vi "transfer char run_subvi_7_25_12c_JW.vi"(0 "VISA session":refnum<visa-resource-name>="GPIB0::17::INSTR", 5 "Var1 sweep settings":T6={"start"=40.0, "stop"=-40.0, "step (linear only)"=-1.0, "sweep spacing (linear: 0)"=0, "sweep mode"=FALSE, "compliance (V)"=100.0, "compliance (A)"=0.001} {"compliance (A)" format="%^.2e"; "compliance (V)" format="%.2f"; "sweep spacing (linear: 0)" items=["linear", "log 10", "log 25", "log 50"]; "step (linear only)" format="%.2f"; "stop" format="%.2f"; "start" format="%.2f"}, 7 "Var2 step settings":T5={"compliance (A)"=0.001, "compliance (V)"=100.0, "start"=-2.0, "total points"=2, "step"=-38.0} {"step" format="%.2f"; "start" format="%.2f"; "compliance (V)" format="%.2f"; "compliance (A)" format="%^.2e"}, 9 "integration time":u32(slide) scale=0.0..2.0, 11 "Input Path":path, 13 "Sample Properties:":T3 {"Date Created" format="%<%x>T"}) -> (2 "Check Cluster":T1, 4 "Output":T2 {"Mobility-Lin" format="%#_4e"; "Mobility-Sat" format="%#_4e"}, 6 "graphic display":cluster{"trace":dbl[], "trace":dbl[]}(graph), 8 "Log Plot":cluster{dbl[], dbl[]}(graph), 10 "XY Graph":cluster{dbl[], "trace":dbl[]}[](graph), 14 "Raw Graph":cluster{dbl[], dbl[]}[](graph), 15 "error?":errorcluster)   [LabVIEW 2011]
uses:
  <vilib>/Utility/file.llb/Write To Spreadsheet File (DBL).vi
panel:
  out "Test Array 2":string[][](array[string])
  out "Test Array":dbl[](array[numeric])
  in  "Output Path":path
  in  "Temp (K)":dbl=0.001 format="%^.2e"
  in  "NumPts":dbl=5.0
  out "Numeric":dbl
  out "min r":dbl
  out "max r":dbl
  out "error? 2":errorcluster
  in  "MAXIMUM":ext format="%.2e"
  in  "MINIMUM":ext=-1e-05 format="%_2e"
  out "graphic display 2":cluster{"trace":dbl[], "trace":dbl[]}(graph)
  in  "Y1 axis":string="Id"
  in  "Y2 axis settings":T4 {"MAXIMUM" format="%.9f"; "MINIMUM" format="%.9f"}
  in  "wait time parameter":dbl=1.0
  in  "Value (Either V or A) 4":dbl
  in  "Value (Either V or A) 3":dbl
  in  "Value (Either V or A) 2":dbl
  in  "Value (V or A)":dbl
  in  "compliance (A)":dbl=0.001 format="%^.2e"
  in  "compliance (V)":dbl=100.0 format="%^.2e"
  in  "Iname":string="Is"
  in  "Vname":string="Vs"
  in  "Function":u16(ring)=4 items=["disabled", "Var1", "Var2", "Var1'", "Constant"]
  in  "Mode":u16(ring)=4 items=["V", "I", "VPulse", "IPulse", "Common"]
  in  "Iname 4":string="I4"
  in  "Vname 4":string="V4"
  in  "Function 4":u16(ring)=4 items=["disabled", "Var1", "Var2", "Var1'", "Constant"]
  in  "Mode 4":u16(ring) items=["V", "I", "VPulse", "IPulse", "Common"]
  in  "Iname 3":string="Ig"
  in  "Vname 3":string="Vg"
  in  "Function 3":u16(ring)=1 items=["disabled", "Var1", "Var2", "Var1'", "Constant"]
  in  "Mode 3":u16(ring) items=["V", "I", "VPulse", "IPulse", "Common"]
  in  "Iname 2":string="Id"
  in  "Vname 2":string="Vd"
  in  "Function 2":u16(ring)=2 items=["disabled", "Var1", "Var2", "Var1'", "Constant"]
  in  "Mode 2":u16(ring) items=["V", "I", "VPulse", "IPulse", "Common"]
  in  "reset":bool=TRUE
  # "SMU1"
  # "SMU2"
  # "SMU3"
  # "SMU4"
  # "Sample Properties:"
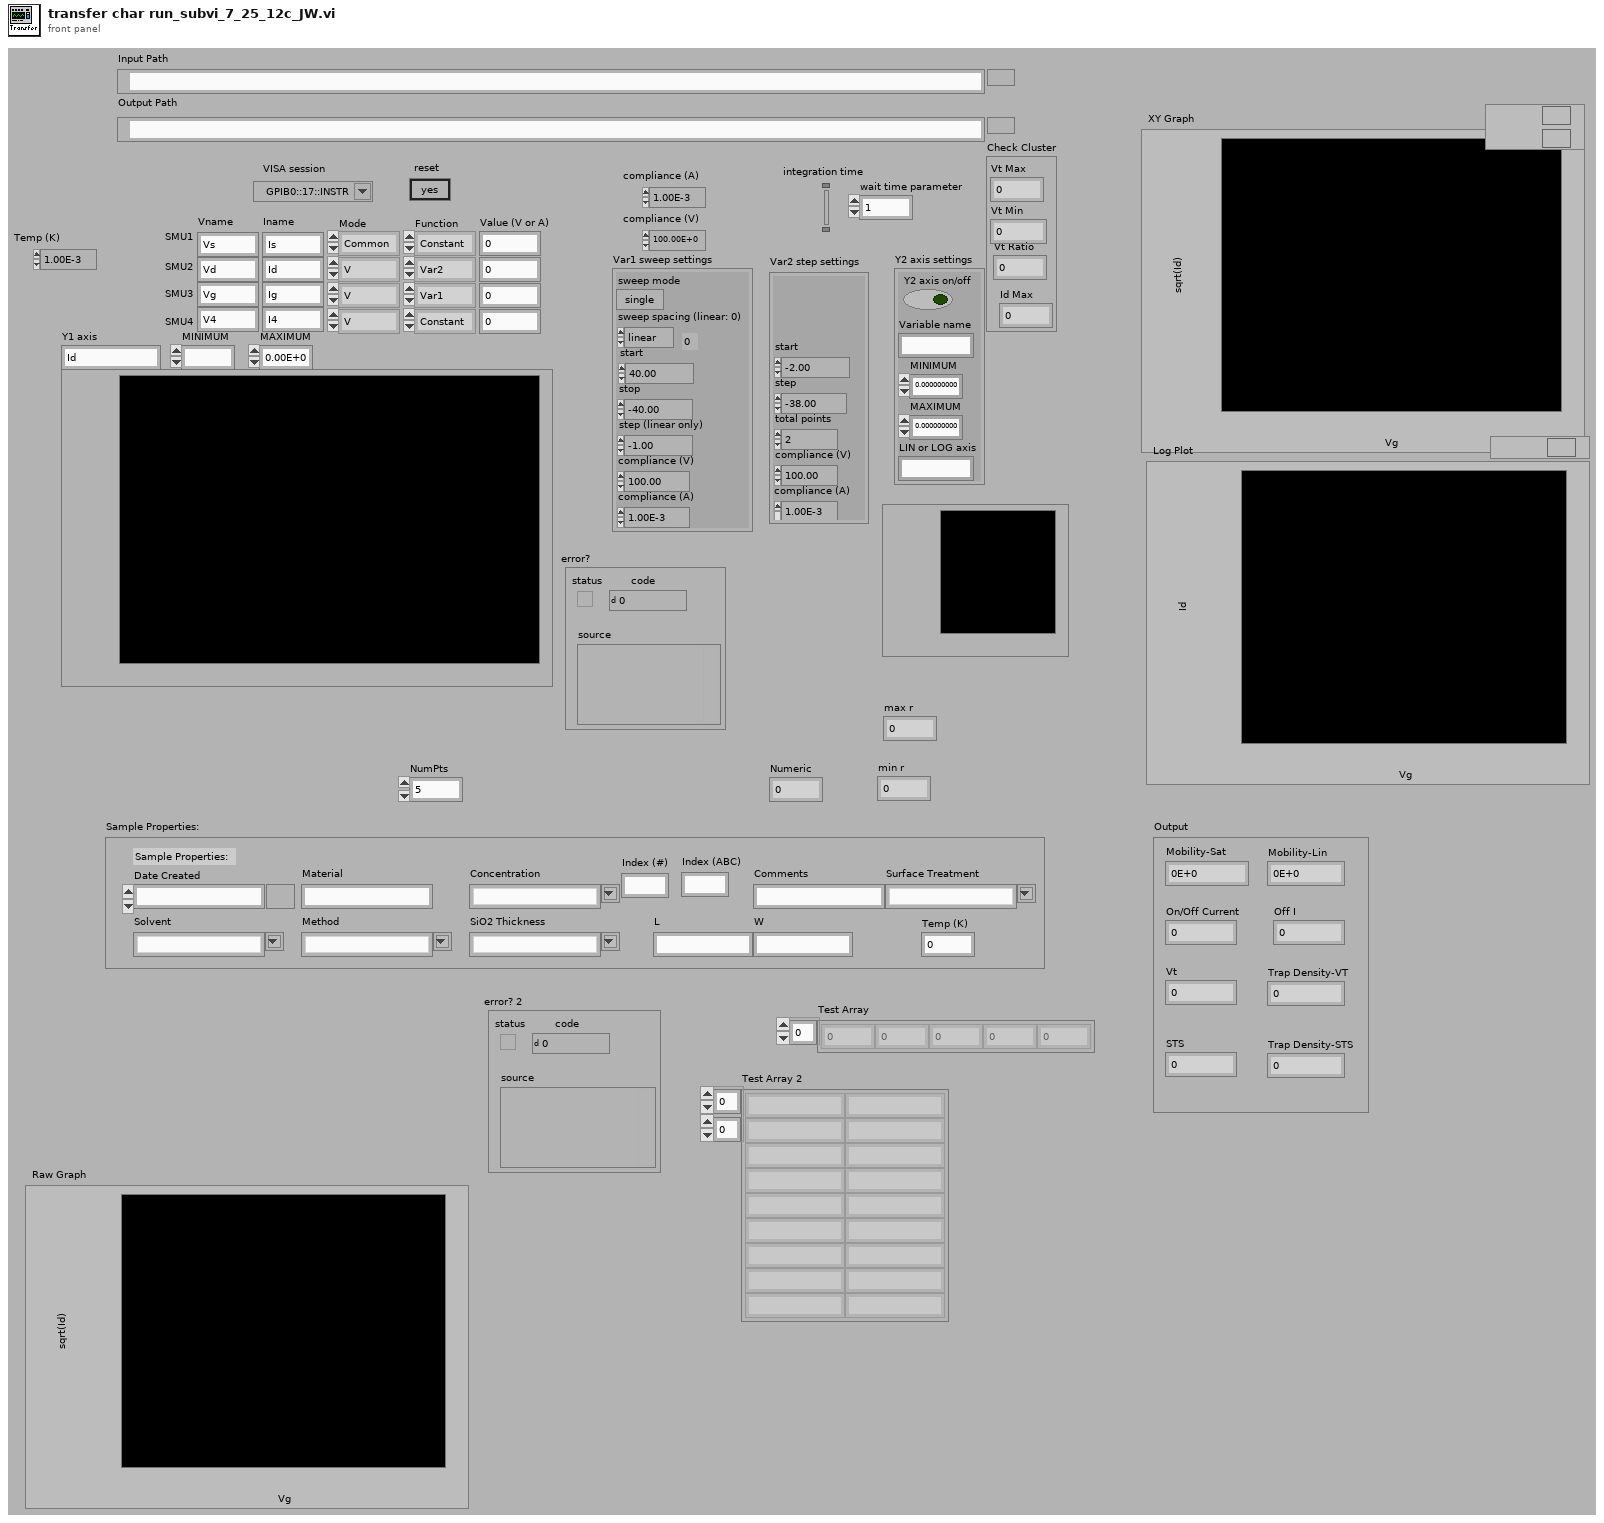
[diagram p1: front panel]
types:
  T1 = cluster{"Vt Max":i32, "Vt Min":i32, "Vt Ratio":i32, "Id Max":dbl}
  T2 = cluster{"Mobility-Sat":dbl, "Mobility-Lin":dbl, "On/Off Current":dbl, "Off I":dbl, "Vt":dbl, "STS":dbl, "Trap Density-VT":dbl, "Trap Density-STS":dbl}
  T3 = cluster{"Date Created":timestamp, "Material":string, "Solvent":string, "Concentration":string, "Method":string, "SiO2 Thickness":string, "Index (#)":string, "Index (ABC)":string, "L":string, "W":string, "Surface Treatment":string, "Comments":string, "Temp (K)":dbl}
  T4 = cluster{"Y2 axis on/off":bool, "MINIMUM":ext, "MAXIMUM":ext, "Variable name":string, "LIN or LOG axis":string}
  T5 = cluster{"compliance (A)":dbl, "compliance (V)":dbl, "start":dbl, "total points":u16, "step":dbl}
  T6 = cluster{"start":dbl, "stop":dbl, "step (linear only)":dbl, "sweep spacing (linear: 0)":u16, "sweep mode":bool, "compliance (V)":dbl, "compliance (A)":dbl}
  T7 = cluster{"Vt Max":dbl, "Vt Min":dbl, "Vt Ratio":dbl, "Id Max":dbl}
  T8 = cluster{"Mobility-Sat":dbl, "Mobility-Lin":dbl, "On/Off I-Sat":dbl, "Off I-Sat":dbl, "VT-Sat":dbl, "Sub Threshold Swing":dbl, "Trap Density-VT":dbl, "Trap Density (N)":dbl}
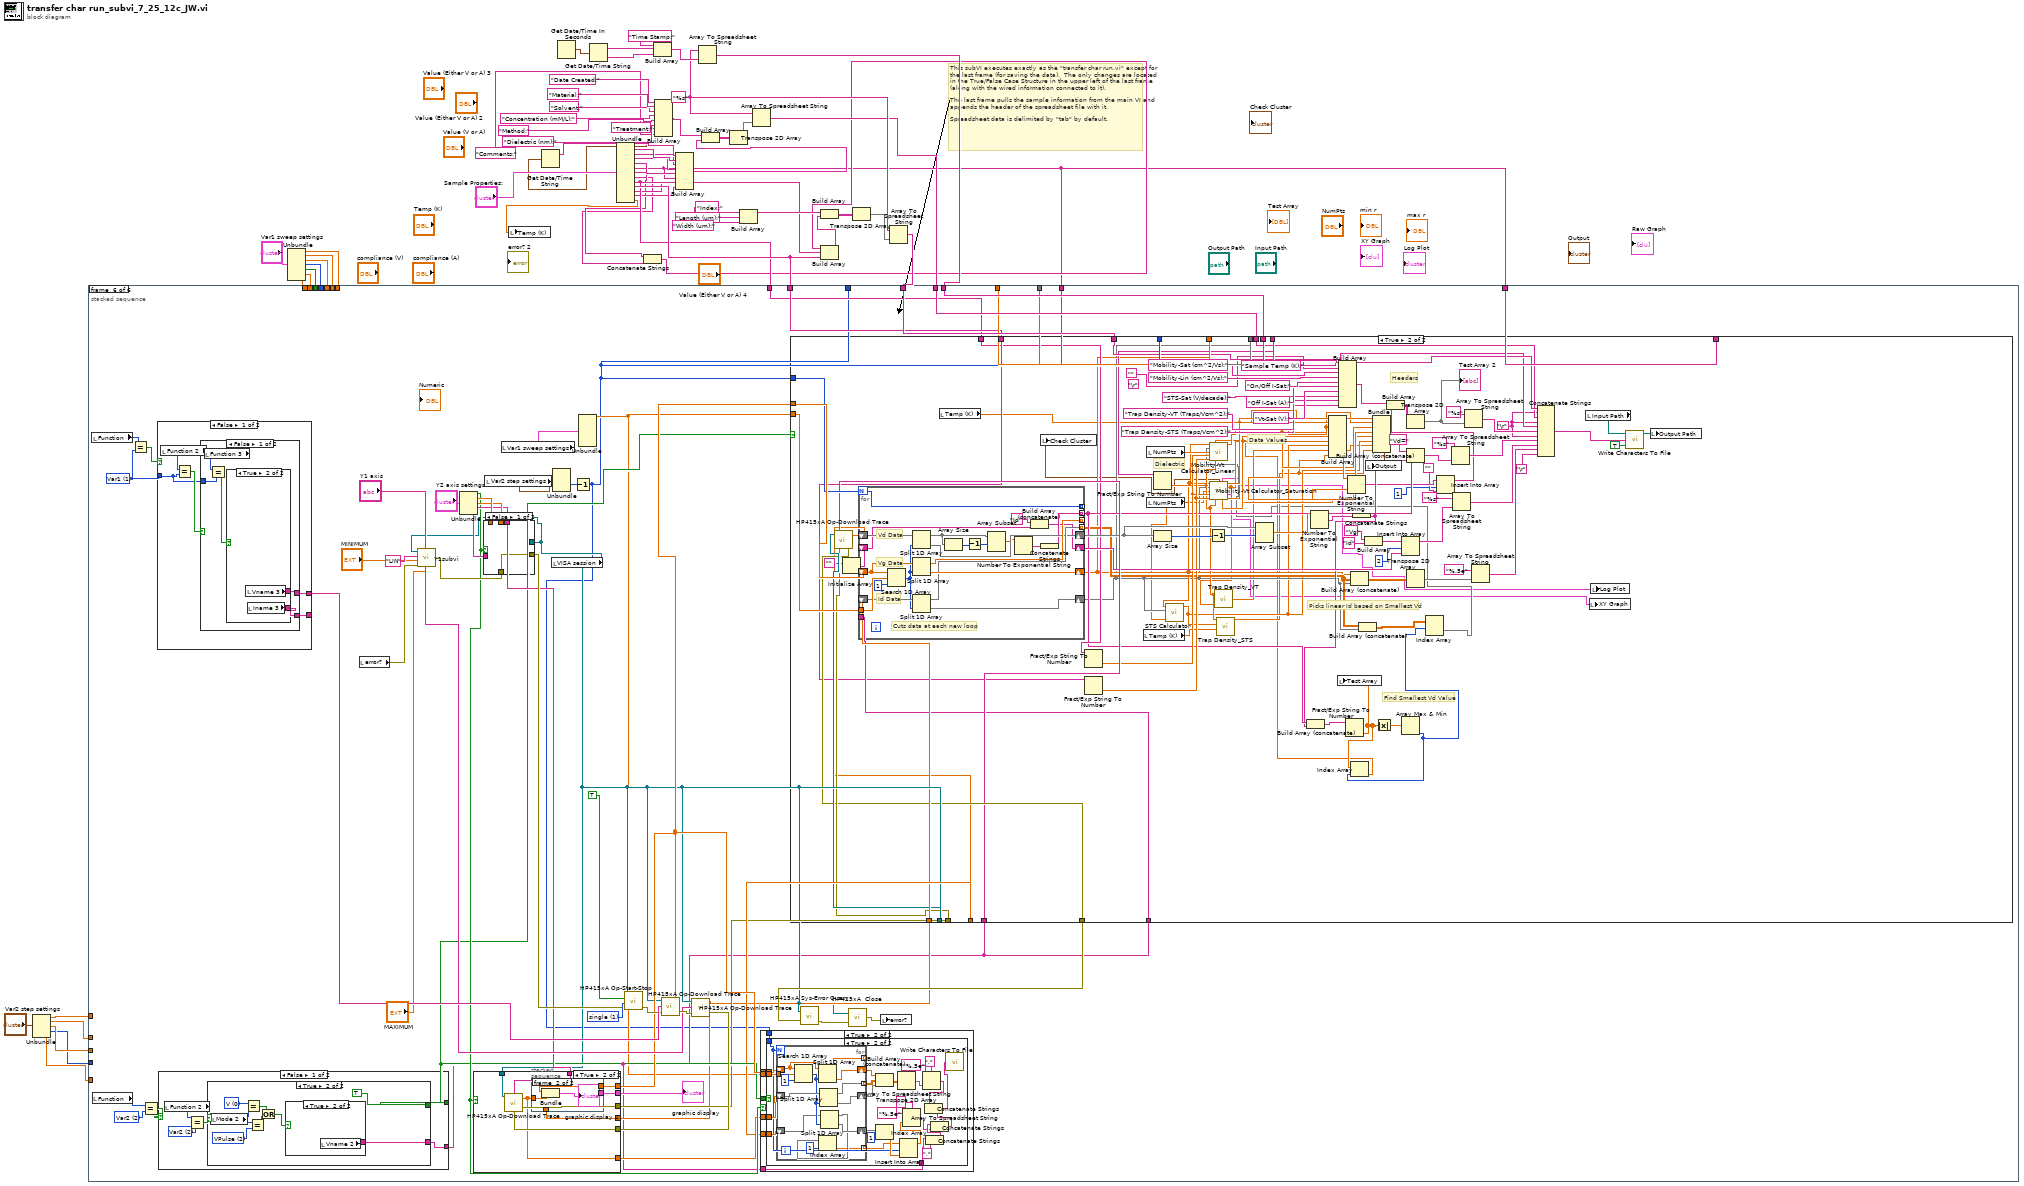
[diagram p0: block diagram]
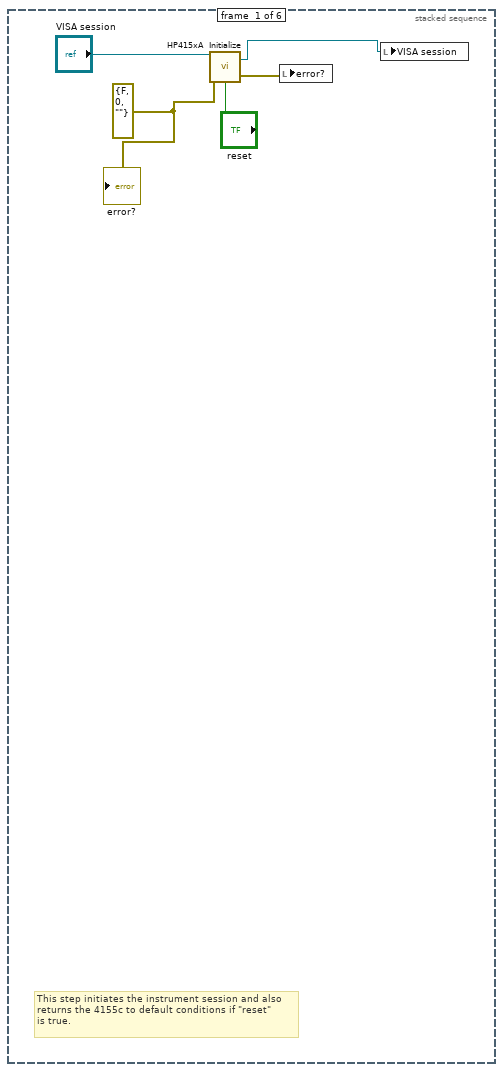
[diagram p2: hidden frame]
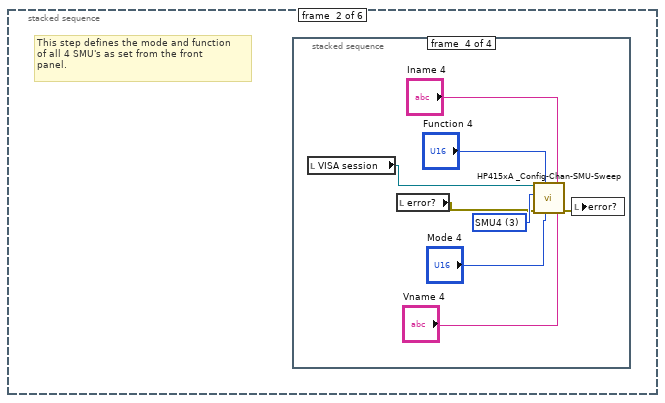
[diagram p3: hidden frame]
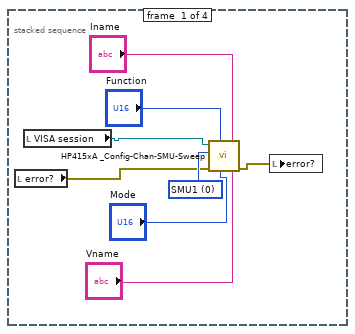
[diagram p4: hidden frame]
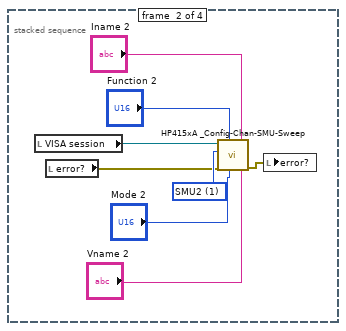
[diagram p5: hidden frame]
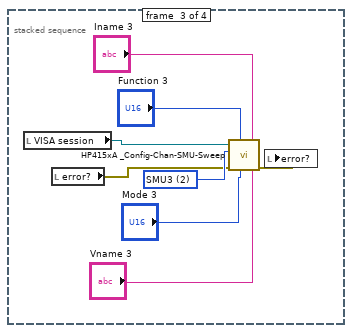
[diagram p6: hidden frame]
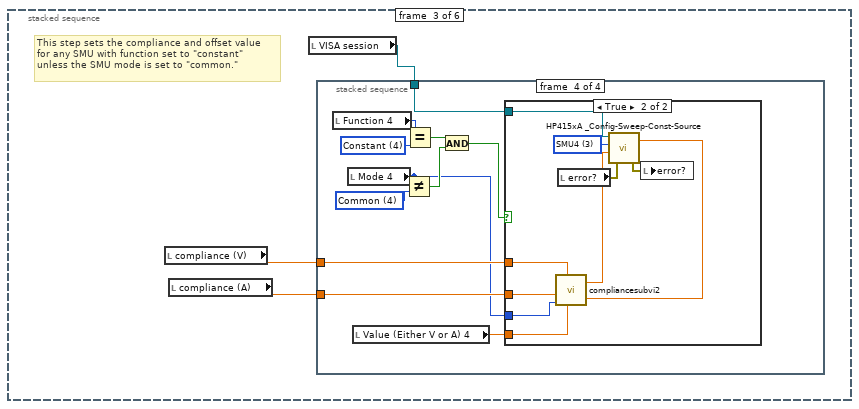
[diagram p7: hidden frame]
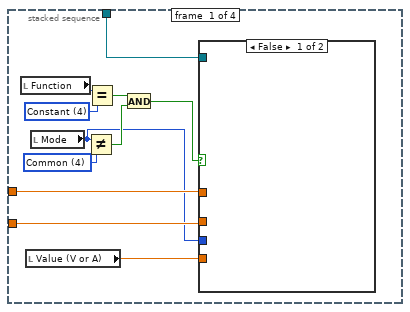
[diagram p8: hidden frame]
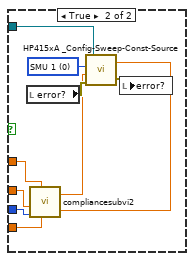
[diagram p9: hidden frame]
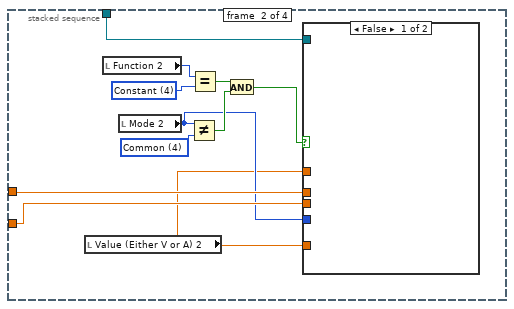
[diagram p10: hidden frame]
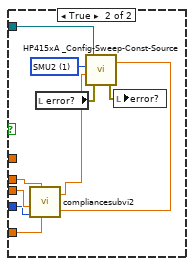
[diagram p11: hidden frame]
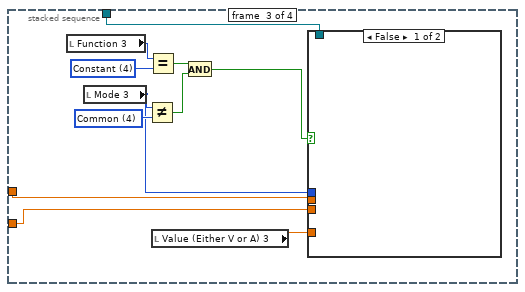
[diagram p12: hidden frame]
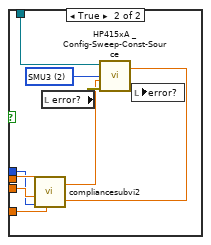
[diagram p13: hidden frame]
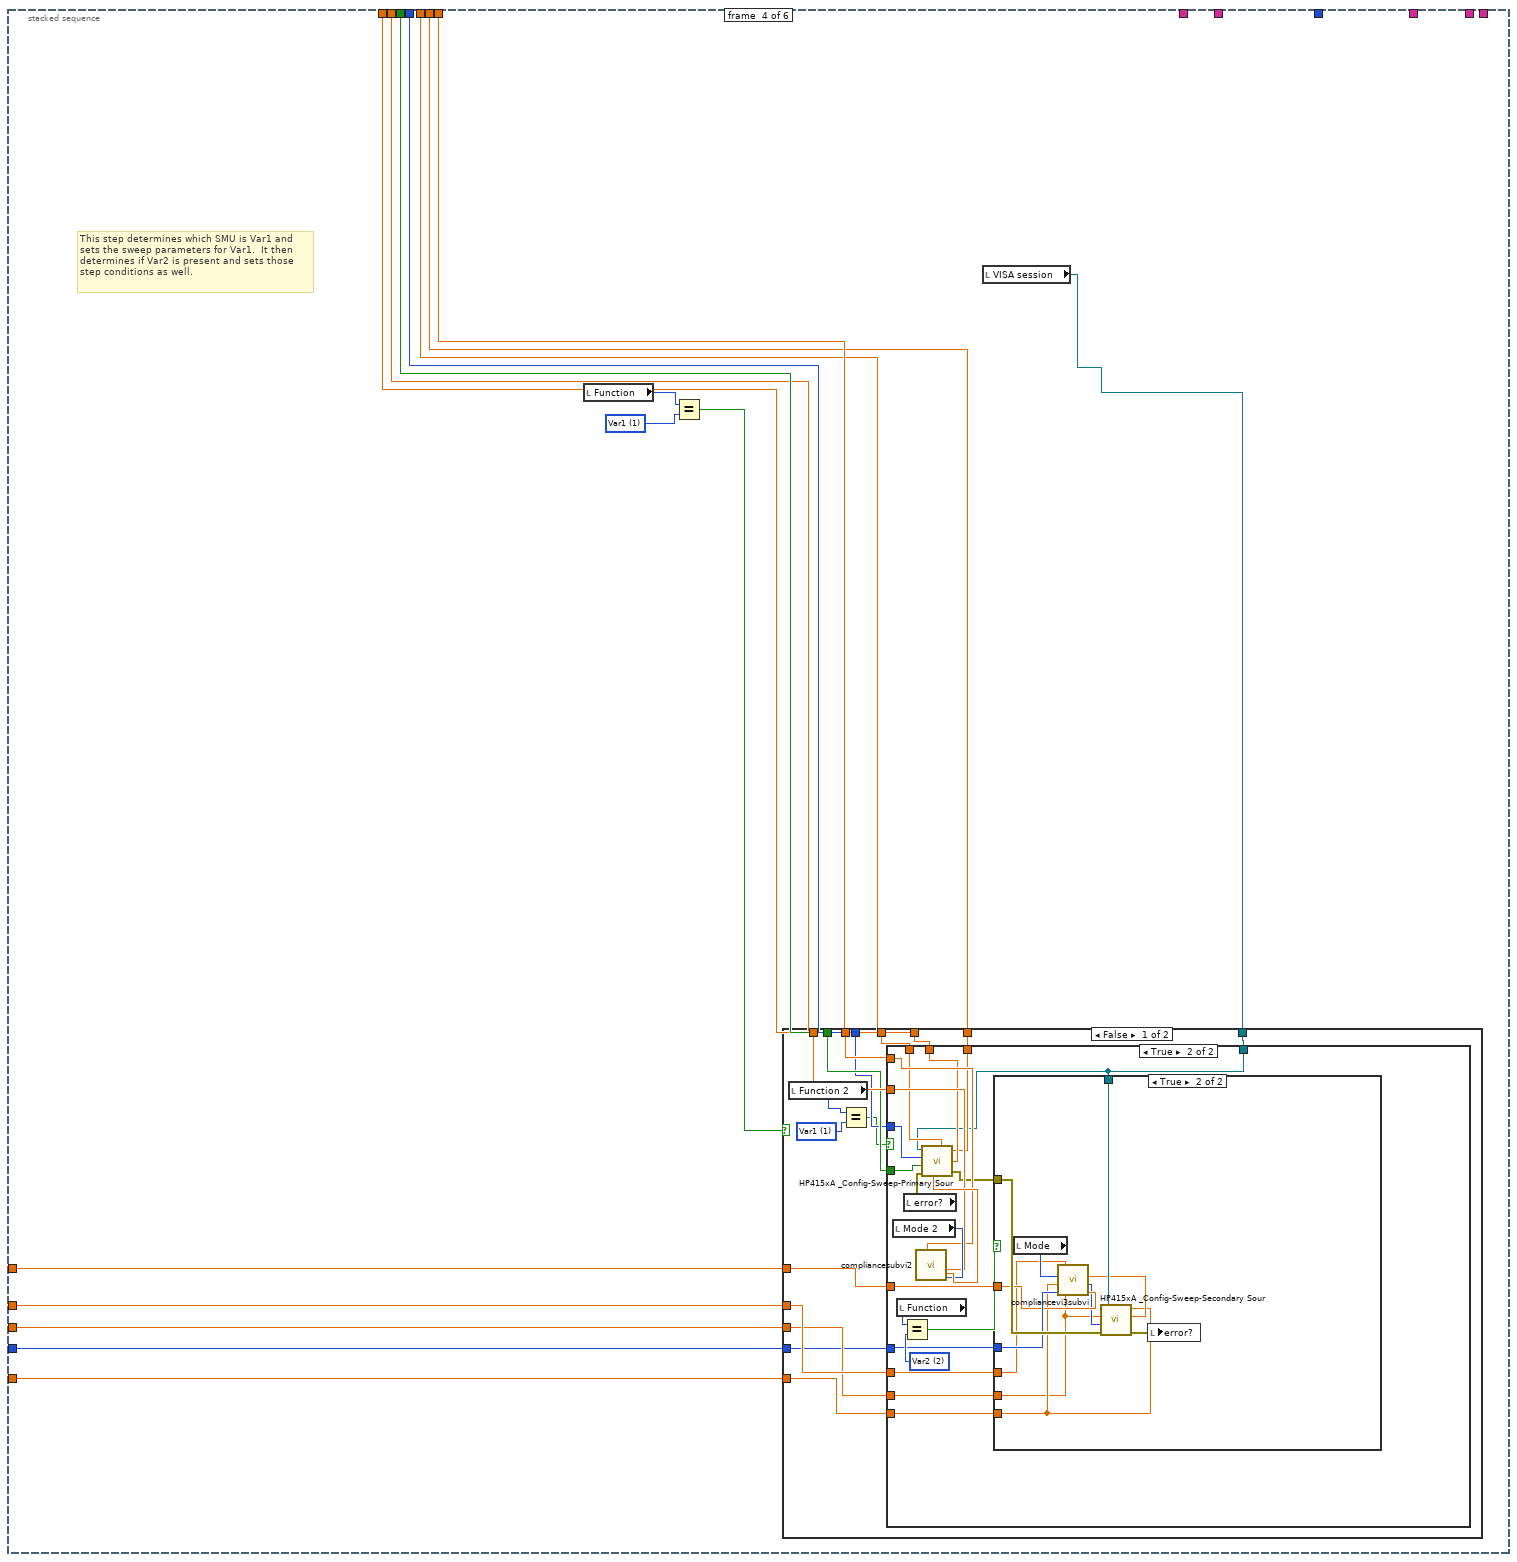
[diagram p15: hidden frame]
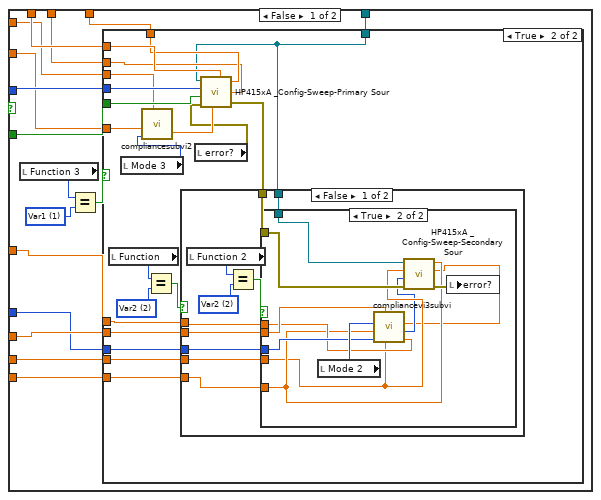
[diagram p16: hidden frame]
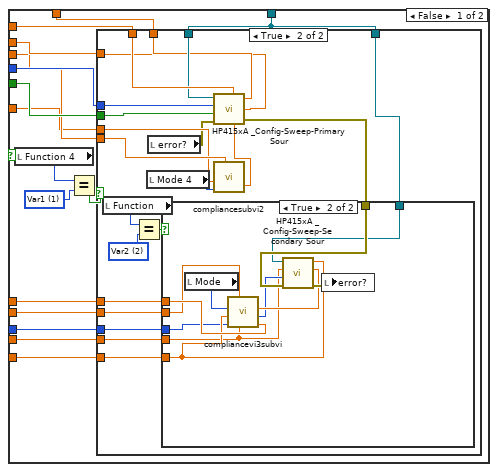
[diagram p17: hidden frame]
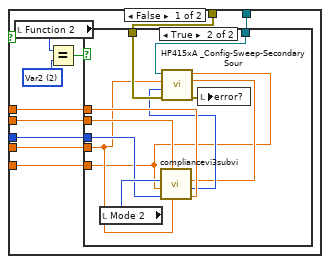
[diagram p19: hidden frame]
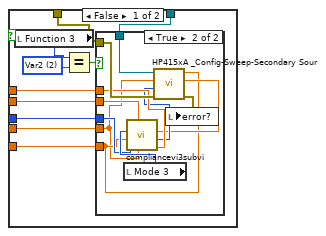
[diagram p20: hidden frame]
diagram:
  w31 = "%s"
  # "This subVI executes exactly as the \"transfer char run.vi\" except for the last frame (for saving the data).  The only changes are located in the True/False Case Structure in the upper left of the last frame (along with the wired information connected to it). \n\nThe last frame pulls the sample information from the main VI and appends the header of the spreadsheet file with it.\n\nSpreadsheet data is delimited by \"tab\" by default."
  n1 = Unbundle("Var2 step settings") -> ("compliance (A)"=w49:dbl, "compliance (V)"=w48:dbl, "start"=w47:dbl, "total points"=w46:u16, "step"=w45:dbl)
  n2 = Unbundle("Var1 sweep settings") -> ("start"=w57:dbl, "stop"=w56:dbl, "step (linear only)"=w55:dbl, "sweep spacing (linear: 0)"=w54:u16, "sweep mode"=w53:bool, "compliance (V)"=w52:dbl, "compliance (A)"=w51:dbl)
  n3 = Get Date/Time In Seconds() -> (seconds since 1Jan1904=w38:timestamp)
  n4 = Get Date/Time String(seconds (now)=w38) -> (date string=w37:string, time string=w36:string)  [unwired: 2 in]
  n5 = Unbundle("Sample Properties:") -> ("Date Created"=w16:timestamp, "Material"=w15:string, "Solvent"=w11:string, "Concentration"=w10:string, "Method"=w14:string, "SiO2 Thickness"=w1:string, "Index (#)"=w5:string, "Index (ABC)"=w4:string, "L"=w8:string, "W"=w9:string, "Surface Treatment"=w7:string, "Comments"=w6:string, "Temp (K)"=w2:dbl)
  n6 = local write "Temp (K)"(w2) -> ()
  n7 = Get Date/Time String(seconds (now)=w16) -> (date string=w43:string)  [unwired: 2 in, 1 out]
  n8 = Concatenate Strings(w5, w4) -> (w3:string)
  n9 = Build Array("Time Stamp:", w37, w36) -> (w35:string[])
  n10 = Build Array("Date Created:", "Material:", "Solvent:", "Concentration (mM/L):", "Method:", "Dielectric (nm):", "Treatment:", "Comments:") -> (w26:string[])
  n11 = Build Array(w43, w15, w11, w10, w14, w1, w7, w6) -> (w25:string[])
  n12 = Array To Spreadsheet String(array=w35, 3:w31) -> (spreadsheet string=w27:string)  [unwired: 1 in]
  n13 = Build Array(w26, w25) -> (w24:string[][])
  n14 = Transpose 2D Array(2D array=w24) -> (transposed array=w23:string[][])
  n15 = Build Array("Index:", "Length (um):", "Width (um):") -> (w22:string[])
  n16 = Array To Spreadsheet String(array=w23, 3:w31) -> (spreadsheet string=w30:string)  [unwired: 1 in]
  n17 = Build Array(w3, w8, w9) -> (w21:string[])
  n18 = Build Array(w22, w21) -> (w20:string[][])
  n19 = Transpose 2D Array(2D array=w20) -> (transposed array=w19:string[][])
  n20 = Array To Spreadsheet String(array=w19, 3:w31) -> (spreadsheet string=w18:string)  [unwired: 1 in]
  n21 = stacked-sequence {
    tunnel: w57 -> [_ _ _ w194 _ _]
    tunnel: w56 -> [_ _ _ w193 _ _]
    tunnel: w55 -> [_ _ _ w192 _ _]
    tunnel: w54 -> [_ _ _ w191 _ _]
    tunnel: w53 -> [_ _ _ w190 _ _]
    tunnel: w52 -> [_ _ _ w189 _ _]
    tunnel: w51 -> [_ _ _ w188 _ _]
    tunnel: w49 -> [_ _ _ w187 _ _]
    tunnel: w48 -> [_ _ _ w186 _ _]
    tunnel: w47 -> [_ _ _ w185 _ _]
    tunnel: w46 -> [_ _ _ w184 _ _]
    tunnel: w45 -> [_ _ _ w183 _ _]
    tunnel: w27 -> [_ _ _ _ _ w558]
    tunnel: w30 -> [_ _ _ _ _ w557]
    tunnel: w18 -> [_ _ _ _ _ w556]
    tunnel: [_ _ _ _ _ w555] -> _
    tunnel: [_ _ _ _ _ w554] -> _
    tunnel: [_ _ _ _ _ w551] -> _
    tunnel: w9 -> [_ _ _ _ _ w553]
    tunnel: w8 -> [_ _ _ _ _ w552]
    tunnel: w1 -> [_ _ _ _ _ w550]
    tunnel: w1 -> [_ _ _ _ _ w549]
    frame #0 {
      w62 = errorcluster {"status"=FALSE, "code"=0, "source"=""} ("error out")
      # "This step initiates the instrument session and also\nreturns the 4155c to default conditions if \"reset\"\nis true."
      n22 = call "HP415xA  Initialize.vi"("instrument descriptor"="VISA session", "reset"="reset", "error in (no error)"=w62) -> ("VISA session"=w59:refnum<visa-resource-name>, "error out"=w61:errorcluster)  [unwired: 2 in]
      n23 = local write "error?"(w61) -> ()
      n24 = local write "VISA session"(w59) -> ()
      "error?" <- w62
    }
    frame #1 {
      # "This step defines the mode and function\nof all 4 SMU's as set from the front\npanel."
      n25 = stacked-sequence {
        frame #0 {
          w71 = u32 0 items=["SMU1  ", "SMU2  ", "SMU3  ", "SMU4  ", "SMU5  ", "SMU6  "] ("unit to configure")
          n26 = local read "error?"() -> (w66:errorcluster)
          n27 = local read "VISA session"() -> (w64:refnum<visa-resource-name>)
          n28 = call "HP415xA _Config-Chan-SMU-Sweep.vi"("V name (max 6 chars)"="Vname", "I name (max 6 chars)"="Iname", "mode"="Mode", "function"="Function", "error in (no error)"=w66, "unit to configure"=w71, "VISA session"=w64) -> ("error out"=w65:errorcluster)  [unwired: 2 in]
          n29 = local write "error?"(w65) -> ()
        }
        frame #1 {
          w75 = u32 1 items=["SMU1  ", "SMU2  ", "SMU3  ", "SMU4  ", "SMU5  ", "SMU6  "] ("unit to configure")
          n30 = local read "VISA session"() -> (w72:refnum<visa-resource-name>)
          n31 = local read "error?"() -> (w73:errorcluster)
          n32 = call "HP415xA _Config-Chan-SMU-Sweep.vi"("V name (max 6 chars)"="Vname 2", "I name (max 6 chars)"="Iname 2", "mode"="Mode 2", "function"="Function 2", "error in (no error)"=w73, "unit to configure"=w75, "VISA session"=w72) -> ("error out"=w74:errorcluster)  [unwired: 2 in]
          n33 = local write "error?"(w74) -> ()
        }
        frame #2 {
          w83 = u32 2 items=["SMU1  ", "SMU2  ", "SMU3  ", "SMU4  ", "SMU5  ", "SMU6  "] ("unit to configure")
          n34 = local read "VISA session"() -> (w80:refnum<visa-resource-name>)
          n35 = local read "error?"() -> (w81:errorcluster)
          n36 = call "HP415xA _Config-Chan-SMU-Sweep.vi"("V name (max 6 chars)"="Vname 3", "I name (max 6 chars)"="Iname 3", "mode"="Mode 3", "function"="Function 3", "error in (no error)"=w81, "unit to configure"=w83, "VISA session"=w80) -> ("error out"=w82:errorcluster)  [unwired: 2 in]
          n37 = local write "error?"(w82) -> ()
        }
        frame #3 {
          w91 = u32 3 items=["SMU1  ", "SMU2  ", "SMU3  ", "SMU4  ", "SMU5  ", "SMU6  "] ("unit to configure")
          n38 = local read "VISA session"() -> (w88:refnum<visa-resource-name>)
          n39 = local read "error?"() -> (w90:errorcluster)
          n40 = call "HP415xA _Config-Chan-SMU-Sweep.vi"("V name (max 6 chars)"="Vname 4", "I name (max 6 chars)"="Iname 4", "mode"="Mode 4", "function"="Function 4", "error in (no error)"=w90, "unit to configure"=w91, "VISA session"=w88) -> ("error out"=w89:errorcluster)  [unwired: 2 in]
          n41 = local write "error?"(w89) -> ()
        }
      }
    }
    frame #2 {
      # "This step sets the compliance and offset value\nfor any SMU with function set to \"constant\"\nunless the SMU mode is set to \"common.\""
      n42 = local read "compliance (V)"() -> (w97:dbl)
      n43 = local read "compliance (A)"() -> (w98:dbl)
      n44 = local read "VISA session"() -> (w96:refnum<visa-resource-name>)
      n45 = stacked-sequence {
        tunnel: w96 -> [w107 w127 w146 w166]
        tunnel: w98 -> [w101 w123 w144 w164]
        tunnel: w97 -> [w100 w122 w143 w165]
        frame #0 {
          w105 = u16 4 items=["V", "I", "VPulse", "IPulse", "Common"] ("Mode")
          w109 = u16 4 items=["disabled", "Var1", "Var2", "Var1'", "Constant"] ("Function")
          n46 = local read "Function"() -> (w108:u16)
          n47 = local read "Value (V or A)"() -> (w102:dbl)
          n48 = local read "Mode"() -> (w99:u16)
          n49 = Not Equal?(x=w99, y=w105) -> (x != y?=w104:bool)
          n50 = Equal?(x=w108, y=w109) -> (x = y?=w106:bool)
          n51 = And(x=w106, y=w104) -> (x .and. y?=w103:bool)
          n52 = case shown="False" w103 {
            tunnel: w107 -> [_ w119]
            tunnel: w100 -> [_ w115]
            tunnel: w101 -> [_ w114]
            tunnel: w102 -> [_ w111]
            tunnel: w99 -> [_ w112]
            frame False {
            }
            frame True {
              w118 = u16 0 items=["SMU 1", "SMU2", "SMU3", "SMU4", "SMU5", "SMU6", "VSU1", "VSU2"] ("unit (SMU1:0)")
              n53 = local read "error?"() -> (w117:errorcluster)
              n54 = call "compliancesubvi2.vi"("Value1"=w111, "compliance (V)"=w115, "Mode"=w112, "compliance (A)"=w114) -> ("compliance"=w113:dbl, "constant"=w110:dbl)  [unwired: 2 in]
              n55 = call "HP415xA _Config-Sweep-Const-Source.vi"("compliance (SMUs only)"=w113, "error in (no error)"=w117, "source (V or A)"=w110, "unit (SMU1:0)"=w118, "VISA session"=w119) -> ("error out"=w116:errorcluster)
              n56 = local write "error?"(w116) -> ()
            }
          }
        }
        frame #1 {
          w124 = u16 4 items=["V", "I", "VPulse", "IPulse", "Common"] ("Mode 2")
          w125 = u16 4 items=["disabled", "Var1", "Var2", "Var1'", "Constant"] ("Function 2")
          n57 = local read "Value (Either V or A) 2"() -> (w120:dbl)
          n58 = local read "Function 2"() -> (w126:u16)
          n59 = local read "Mode 2"() -> (w121:u16)
          n60 = Not Equal?(x=w121, y=w124) -> (x != y?=w129:bool)
          n61 = Equal?(x=w126, y=w125) -> (x = y?=w130:bool)
          n62 = And(x=w130, y=w129) -> (x .and. y?=w128:bool)
          n63 = case shown="False" w128 {
            tunnel: w127 -> [_ w140]
            tunnel: w122 -> [_ w138]
            tunnel: w123 -> [_ w137]
            tunnel: w120 -> [_ _]
            tunnel: w121 -> [_ w133]
            tunnel: w120 -> [_ w132]
            frame False {
            }
            frame True {
              w139 = u16 1 items=["SMU 1", "SMU2", "SMU3", "SMU4", "SMU5", "SMU6", "VSU1", "VSU2"] ("unit (SMU1:0)")
              n64 = call "compliancesubvi2.vi"("Value1"=w132, "compliance (V)"=w138, "Mode"=w133, "compliance (A)"=w137) -> ("compliance"=w136:dbl, "constant"=w131:dbl)  [unwired: 2 in]
              n65 = local read "error?"() -> (w135:errorcluster)
              n66 = call "HP415xA _Config-Sweep-Const-Source.vi"("compliance (SMUs only)"=w136, "error in (no error)"=w135, "source (V or A)"=w131, "unit (SMU1:0)"=w139, "VISA session"=w140) -> ("error out"=w134:errorcluster)
              n67 = local write "error?"(w134) -> ()
            }
          }
        }
        frame #2 {
          w148 = u16 4 items=["V", "I", "VPulse", "IPulse", "Common"] ("Mode 2")
          w149 = u16 4 items=["disabled", "Var1", "Var2", "Var1'", "Constant"] ("Function 2")
          n68 = local read "Function 3"() -> (w147:u16)
          n69 = local read "Mode 3"() -> (w142:u16)
          n70 = Not Equal?(x=w142, y=w148) -> (x != y?=w150:bool)
          n71 = Equal?(x=w147, y=w149) -> (x = y?=w151:bool)
          n72 = local read "Value (Either V or A) 3"() -> (w145:dbl)
          n73 = And(x=w151, y=w150) -> (x .and. y?=w141:bool)
          n74 = case shown="False" w141 {
            tunnel: w146 -> [_ w159]
            tunnel: w145 -> [_ w153]
            tunnel: w144 -> [_ w156]
            tunnel: w143 -> [_ w155]
            tunnel: w142 -> [_ w154]
            frame False {
            }
            frame True {
              w158 = u16 2 items=["SMU 1", "SMU2", "SMU3", "SMU4", "SMU5", "SMU6", "VSU1", "VSU2"] ("unit (SMU1:0)")
              n75 = call "compliancesubvi2.vi"("Value1"=w153, "compliance (V)"=w155, "Mode"=w154, "compliance (A)"=w156) -> ("compliance"=w157:dbl, "constant"=w152:dbl)  [unwired: 2 in]
              n76 = local read "error?"() -> (w161:errorcluster)
              n77 = call "HP415xA _Config-Sweep-Const-Source.vi"("compliance (SMUs only)"=w157, "error in (no error)"=w161, "source (V or A)"=w152, "unit (SMU1:0)"=w158, "VISA session"=w159) -> ("error out"=w160:errorcluster)
              n78 = local write "error?"(w160) -> ()
            }
          }
        }
        frame #3 {
          w168 = u16 4 items=["V", "I", "VPulse", "IPulse", "Common"] ("Mode 4")
          w169 = u16 4 items=["disabled", "Var1", "Var2", "Var1'", "Constant"] ("Function 4")
          n79 = local read "Function 4"() -> (w170:u16)
          n80 = local read "Mode 4"() -> (w163:u16)
          n81 = local read "Value (Either V or A) 4"() -> (w162:dbl)
          n82 = Not Equal?(x=w163, y=w168) -> (x != y?=w171:bool)
          n83 = Equal?(x=w170, y=w169) -> (x = y?=w172:bool)
          n84 = And(x=w172, y=w171) -> (x .and. y?=w167:bool)
          n85 = case shown="True" w167 {
            tunnel: w166 -> [_ w181]
            tunnel: w165 -> [_ w177]
            tunnel: w164 -> [_ w178]
            tunnel: w163 -> [_ w176]
            tunnel: w162 -> [_ w175]
            frame False {
            }
            frame True {
              w182 = u16 3 items=["SMU 1", "SMU2", "SMU3", "SMU4", "SMU5", "SMU6", "VSU1", "VSU2"] ("unit (SMU1:0)")
              n86 = call "compliancesubvi2.vi"("Value1"=w175, "compliance (V)"=w177, "Mode"=w176, "compliance (A)"=w178) -> ("compliance"=w174:dbl, "constant"=w173:dbl)  [unwired: 2 in]
              n87 = local read "error?"() -> (w180:errorcluster)
              n88 = call "HP415xA _Config-Sweep-Const-Source.vi"("compliance (SMUs only)"=w174, "error in (no error)"=w180, "source (V or A)"=w173, "unit (SMU1:0)"=w182, "VISA session"=w181) -> ("error out"=w179:errorcluster)
              n89 = local write "error?"(w179) -> ()
            }
          }
        }
      }
    }
    frame #3 {
      w198 = u16 1 items=["disabled", "Var1", "Var2", "Var1'", "Constant"] ("Function")
      # "This step determines which SMU is Var1 and\nsets the sweep parameters for Var1.  It then\ndetermines if Var2 is present and sets those\nstep conditions as well."
      n90 = local read "Function"() -> (w197:u16)
      n91 = Equal?(x=w197, y=w198) -> (x = y?=w196:bool)
      n92 = local read "VISA session"() -> (w195:refnum<visa-resource-name>)
      n93 = case shown="False" w196 {
        tunnel: w189 -> [w211 w487]
        tunnel: w188 -> [w212 w486]
        tunnel: w191 -> [w209 w485]
        tunnel: w190 -> [w210 w484]
        tunnel: w192 -> [w206 w483]
        tunnel: w193 -> [w205 w482]
        tunnel: w194 -> [w207 w481]
        tunnel: w195 -> [w208 w470]
        tunnel: w187 -> [w203 w476]
        tunnel: w186 -> [w202 w475]
        tunnel: w185 -> [w201 w474]
        tunnel: w184 -> [w200 w473]
        tunnel: w183 -> [w199 w472]
        frame False {
          w214 = u16 1 items=["disabled", "Var1", "Var2", "Var1'", "Constant"] ("Function")
          n94 = local read "Function 2"() -> (w213:u16)
          n95 = Equal?(x=w213, y=w214) -> (x = y?=w204:bool)
          n96 = case shown="True" w204 {
            tunnel: w212 -> [w220 w413]
            tunnel: w211 -> [w221 w412]
            tunnel: w210 -> [w222 w411]
            tunnel: w209 -> [w223 w410]
            tunnel: w208 -> [w227 w399]
            tunnel: w207 -> [w226 w409]
            tunnel: w206 -> [w224 w408]
            tunnel: w205 -> [w225 w407]
            tunnel: w203 -> [w219 w402]
            tunnel: w202 -> [w218 w401]
            tunnel: w201 -> [w216 w400]
            tunnel: w200 -> [w217 w397]
            tunnel: w199 -> [w215 w396]
            frame False {
              w230 = u16 1 items=["disabled", "Var1", "Var2", "Var1'", "Constant"] ("Function")
              n97 = local read "Function 3"() -> (w229:u16)
              n98 = Equal?(x=w229, y=w230) -> (x = y?=w228:bool)
              n99 = case shown="True" w228 {
                tunnel: w227 -> [w231 w324]
                tunnel: w226 -> [w243 w341]
                tunnel: w225 -> [w240 w340]
                tunnel: w224 -> [w239 w339]
                tunnel: w223 -> [w242 w338]
                tunnel: w222 -> [w241 w337]
                tunnel: w221 -> [w238 w336]
                tunnel: w220 -> [w237 w335]
                tunnel: w219 -> [w236 w328]
                tunnel: w218 -> [w235 w327]
                tunnel: w217 -> [w234 w326]
                tunnel: w216 -> [w233 w323]
                tunnel: w215 -> [w232 w322]
                frame False {
                  w246 = u16 1 items=["disabled", "Var1", "Var2", "Var1'", "Constant"] ("Function")
                  n100 = local read "Function 4"() -> (w245:u16)
                  n101 = Equal?(x=w245, y=w246) -> (x = y?=w244:bool)
                  n102 = case shown="True" w244 {
                    tunnel: w243 -> [_ w265]
                    tunnel: w231 -> [_ w264]
                    tunnel: w242 -> [_ w263]
                    tunnel: w241 -> [_ w262]
                    tunnel: w240 -> [_ w261]
                    tunnel: w239 -> [_ w260]
                    tunnel: w238 -> [_ w259]
                    tunnel: w237 -> [_ w258]
                    tunnel: w236 -> [_ w253]
                    tunnel: w235 -> [_ w252]
                    tunnel: w234 -> [_ w251]
                    tunnel: w233 -> [_ w250]
                    tunnel: w232 -> [_ w249]
                    tunnel: w231 -> [_ w247]
                    frame False {
                    }
                    frame True {
                      w256 = u16 2 items=["disabled", "Var1", "Var2", "Var1'", "Constant"] ("Function")
                      n103 = local read "Function"() -> (w255:u16)
                      n104 = Equal?(x=w255, y=w256) -> (x = y?=w254:bool)
                      n105 = local read "Mode 4"() -> (w267:u16)
                      n106 = local read "error?"() -> (w257:errorcluster)
                      n107 = call "compliancesubvi2.vi"("compliance (V)"=w259, "Mode"=w267, "compliance (A)"=w258) -> ("compliance"=w266:dbl)  [unwired: 3 in, 1 out]
                      n108 = call "HP415xA _Config-Sweep-Primary Sour.vi"("step (linear only)"=w260, "stop"=w261, "start"=w265, "compliance"=w266, "error in (no error)"=w257, "sweep mode"=w262, "sweep spacing (linear: 0)"=w263, "VISA session"=w264) -> ("error out"=w248:errorcluster)  [unwired: 2 in]
                      n109 = case shown="True" w254 {
                        tunnel: w253 -> [w274 w317]
                        tunnel: w252 -> [w273 w312]
                        tunnel: w251 -> [w272 w311]
                        tunnel: w250 -> [w271 w313]
                        tunnel: w249 -> [w270 w316]
                        tunnel: w248 -> [w269 w319]
                        tunnel: w247 -> [w268 w318]
                        frame False {
                          w277 = u16 2 items=["disabled", "Var1", "Var2", "Var1'", "Constant"] ("Function")
                          n110 = local read "Function 2"() -> (w276:u16)
                          n111 = Equal?(x=w276, y=w277) -> (x = y?=w275:bool)
                          n112 = case shown="True" w275 {
                            tunnel: w274 -> [w285 w305]
                            tunnel: w273 -> [w284 w306]
                            tunnel: w272 -> [w283 w304]
                            tunnel: w271 -> [w282 w302]
                            tunnel: w270 -> [w281 w300]
                            tunnel: w269 -> [w280 w310]
                            tunnel: w268 -> [w278 w309]
                            frame False {
                              w287 = u16 2 items=["disabled", "Var1", "Var2", "Var1'", "Constant"] ("Function")
                              n113 = local read "Function 3"() -> (w279:u16)
                              n114 = Equal?(x=w279, y=w287) -> (x = y?=w286:bool)
                              n115 = case shown="True" w286 {
                                tunnel: w285 -> [_ w293]
                                tunnel: w284 -> [_ w294]
                                tunnel: w283 -> [_ w295]
                                tunnel: w282 -> [_ w289]
                                tunnel: w281 -> [_ w290]
                                tunnel: w280 -> [w288 w299]
                                tunnel: w278 -> [_ w298]
                                frame False {
                                n116 = local write "error?"(w288) -> ()
                                }
                                frame True {
                                n117 = local read "Mode 3"() -> (w297:u16)
                                n118 = call "compliancevi3subvi.vi"("compliance (A)"=w293, "start"=w289, "compliance (V)"=w294, "total points"=w295, "step"=w290, "Mode"=w297) -> ("total points 2"=w292:u16, "compliance"=w291:dbl)  [unwired: 1 in, 1 out]
                                n119 = call "HP415xA _Config-Sweep-Secondary Sour.vi"("compliance"=w291, "step"=w290, "error in (no error)"=w299, "total points"=w292, "start"=w289, "VISA session"=w298) -> ("error out"=w296:errorcluster)  [unwired: 1 in]
                                n120 = local write "error?"(w296) -> ()
                                }
                              }
                            }
                            frame True {
                              n121 = local read "Mode 2"() -> (w308:u16)
                              n122 = call "compliancevi3subvi.vi"("compliance (A)"=w305, "start"=w302, "compliance (V)"=w306, "total points"=w304, "step"=w300, "Mode"=w308) -> ("total points 2"=w303:u16, "compliance"=w301:dbl)  [unwired: 1 in, 1 out]
                              n123 = call "HP415xA _Config-Sweep-Secondary Sour.vi"("compliance"=w301, "step"=w300, "error in (no error)"=w310, "total points"=w303, "start"=w302, "VISA session"=w309) -> ("error out"=w307:errorcluster)  [unwired: 1 in]
                              n124 = local write "error?"(w307) -> ()
                            }
                          }
                        }
                        frame True {
                          n125 = local read "Mode"() -> (w321:u16)
                          n126 = call "compliancevi3subvi.vi"("compliance (A)"=w317, "start"=w313, "compliance (V)"=w312, "total points"=w311, "step"=w316, "Mode"=w321) -> ("total points 2"=w314:u16, "compliance"=w315:dbl)  [unwired: 1 in, 1 out]
                          n127 = call "HP415xA _Config-Sweep-Secondary Sour.vi"("compliance"=w315, "step"=w316, "error in (no error)"=w319, "total points"=w314, "start"=w313, "VISA session"=w318) -> ("error out"=w320:errorcluster)  [unwired: 1 in]
                          n128 = local write "error?"(w320) -> ()
                        }
                      }
                    }
                  }
                }
                frame True {
                  w331 = u16 2 items=["disabled", "Var1", "Var2", "Var1'", "Constant"] ("Function")
                  n129 = local read "Function"() -> (w330:u16)
                  n130 = local read "Mode 3"() -> (w333:u16)
                  n131 = call "compliancesubvi2.vi"("compliance (V)"=w336, "Mode"=w333, "compliance (A)"=w335) -> ("compliance"=w334:dbl)  [unwired: 3 in, 1 out]
                  n132 = Equal?(x=w330, y=w331) -> (x = y?=w329:bool)
                  n133 = local read "error?"() -> (w332:errorcluster)
                  n134 = call "HP415xA _Config-Sweep-Primary Sour.vi"("step (linear only)"=w339, "stop"=w340, "start"=w341, "compliance"=w334, "error in (no error)"=w332, "sweep mode"=w337, "sweep spacing (linear: 0)"=w338, "VISA session"=w324) -> ("error out"=w325:errorcluster)  [unwired: 2 in]
                  n135 = case shown="False" w329 {
                    tunnel: w328 -> [w346 w391]
                    tunnel: w327 -> [w345 w390]
                    tunnel: w326 -> [w343 w389]
                    tunnel: w325 -> [w348 w394]
                    tunnel: w324 -> [w347 w393]
                    tunnel: w323 -> [w342 w386]
                    tunnel: w322 -> [w344 w385]
                    frame False {
                      w351 = u16 2 items=["disabled", "Var1", "Var2", "Var1'", "Constant"] ("Function")
                      n136 = local read "Function 2"() -> (w350:u16)
                      n137 = Equal?(x=w350, y=w351) -> (x = y?=w349:bool)
                      n138 = case shown="True" w349 {
                        tunnel: w348 -> [w358 w383]
                        tunnel: w347 -> [w357 w382]
                        tunnel: w346 -> [w356 w378]
                        tunnel: w345 -> [w355 w379]
                        tunnel: w344 -> [w352 w377]
                        tunnel: w343 -> [w354 w380]
                        tunnel: w342 -> [w353 w376]
                        frame False {
                          w361 = u16 2 items=["disabled", "Var1", "Var2", "Var1'", "Constant"] ("Function")
                          n139 = local read "Function 4"() -> (w360:u16)
                          n140 = Equal?(x=w360, y=w361) -> (x = y?=w359:bool)
                          n141 = case shown="True" w359 {
                            tunnel: w358 -> [w362 w371]
                            tunnel: w357 -> [_ w372]
                            tunnel: w356 -> [_ w368]
                            tunnel: w355 -> [_ w369]
                            tunnel: w354 -> [_ w367]
                            tunnel: w353 -> [_ w364]
                            tunnel: w352 -> [_ w363]
                            frame False {
                              n142 = local write "error?"(w362) -> ()
                            }
                            frame True {
                              n143 = local read "Mode 4"() -> (w373:u16)
                              n144 = call "compliancevi3subvi.vi"("compliance (A)"=w368, "start"=w364, "compliance (V)"=w369, "total points"=w367, "step"=w363, "Mode"=w373) -> ("total points 2"=w366:u16, "compliance"=w365:dbl)  [unwired: 1 in, 1 out]
                              n145 = call "HP415xA _Config-Sweep-Secondary Sour.vi"("compliance"=w365, "step"=w363, "error in (no error)"=w371, "total points"=w366, "start"=w364, "VISA session"=w372) -> ("error out"=w370:errorcluster)  [unwired: 1 in]
                              n146 = local write "error?"(w370) -> ()
                            }
                          }
                        }
                        frame True {
                          n147 = local read "Mode 2"() -> (w384:u16)
                          n148 = call "compliancevi3subvi.vi"("compliance (A)"=w378, "start"=w376, "compliance (V)"=w379, "total points"=w380, "step"=w377, "Mode"=w384) -> ("total points 2"=w375:u16, "compliance"=w374:dbl)  [unwired: 1 in, 1 out]
                          n149 = call "HP415xA _Config-Sweep-Secondary Sour.vi"("compliance"=w374, "step"=w377, "error in (no error)"=w383, "total points"=w375, "start"=w376, "VISA session"=w382) -> ("error out"=w381:errorcluster)  [unwired: 1 in]
                          n150 = local write "error?"(w381) -> ()
                        }
                      }
                    }
                    frame True {
                      n151 = local read "Mode"() -> (w395:u16)
                      n152 = call "compliancevi3subvi.vi"("compliance (A)"=w391, "start"=w386, "compliance (V)"=w390, "total points"=w389, "step"=w385, "Mode"=w395) -> ("total points 2"=w388:u16, "compliance"=w387:dbl)  [unwired: 1 in, 1 out]
                      n153 = call "HP415xA _Config-Sweep-Secondary Sour.vi"("compliance"=w387, "step"=w385, "error in (no error)"=w394, "total points"=w388, "start"=w386, "VISA session"=w393) -> ("error out"=w392:errorcluster)  [unwired: 1 in]
                      n154 = local write "error?"(w392) -> ()
                    }
                  }
                }
              }
            }
            frame True {
              w405 = u16 2 items=["disabled", "Var1", "Var2", "Var1'", "Constant"] ("Function")
              n155 = local read "Mode 2"() -> (w414:u16)
              n156 = local read "Function"() -> (w404:u16)
              n157 = Equal?(x=w404, y=w405) -> (x = y?=w403:bool)
              n158 = local read "error?"() -> (w406:errorcluster)
              n159 = call "compliancesubvi2.vi"("compliance (V)"=w412, "Mode"=w414, "compliance (A)"=w413) -> ("compliance"=w415:dbl)  [unwired: 3 in, 1 out]
              n160 = call "HP415xA _Config-Sweep-Primary Sour.vi"("step (linear only)"=w408, "stop"=w407, "start"=w409, "compliance"=w415, "error in (no error)"=w406, "sweep mode"=w411, "sweep spacing (linear: 0)"=w410, "VISA session"=w399) -> ("error out"=w398:errorcluster)  [unwired: 2 in]
              n161 = case shown="True" w403 {
                tunnel: w402 -> [w421 w464]
                tunnel: w401 -> [w420 w463]
                tunnel: w400 -> [w418 w459]
                tunnel: w399 -> [w423 w469]
                tunnel: w398 -> [w417 w468]
                tunnel: w397 -> [w419 w465]
                tunnel: w396 -> [w416 w461]
                frame False {
                  w425 = u16 2 items=["disabled", "Var1", "Var2", "Var1'", "Constant"] ("Function")
                  n162 = local read "Function 3"() -> (w424:u16)
                  n163 = Equal?(x=w424, y=w425) -> (x = y?=w422:bool)
                  n164 = case shown="True" w422 {
                    tunnel: w423 -> [w431 w457]
                    tunnel: w421 -> [w430 w454]
                    tunnel: w420 -> [w428 w452]
                    tunnel: w419 -> [w429 w453]
                    tunnel: w418 -> [w426 w450]
                    tunnel: w417 -> [w432 w456]
                    tunnel: w416 -> [w427 w448]
                    frame False {
                      w435 = u16 2 items=["disabled", "Var1", "Var2", "Var1'", "Constant"] ("Function")
                      n165 = local read "Function 4"() -> (w434:u16)
                      n166 = Equal?(x=w434, y=w435) -> (x = y?=w433:bool)
                      n167 = case shown="True" w433 {
                        tunnel: w432 -> [w436 w447]
                        tunnel: w431 -> [_ w446]
                        tunnel: w430 -> [_ w443]
                        tunnel: w429 -> [_ w444]
                        tunnel: w428 -> [_ w442]
                        tunnel: w427 -> [_ w438]
                        tunnel: w426 -> [_ w439]
                        frame False {
                          n168 = local write "error?"(w436) -> ()
                        }
                        frame True {
                          n169 = local read "Mode 4"() -> (w441:u16)
                          n170 = call "compliancevi3subvi.vi"("compliance (A)"=w443, "start"=w439, "compliance (V)"=w442, "total points"=w444, "step"=w438, "Mode"=w441) -> ("total points 2"=w440:u16, "compliance"=w437:dbl)  [unwired: 1 in, 1 out]
                          n171 = call "HP415xA _Config-Sweep-Secondary Sour.vi"("compliance"=w437, "step"=w438, "error in (no error)"=w447, "total points"=w440, "start"=w439, "VISA session"=w446) -> ("error out"=w445:errorcluster)  [unwired: 1 in]
                          n172 = local write "error?"(w445) -> ()
                        }
                      }
                    }
                    frame True {
                      n173 = local read "Mode 3"() -> (w458:u16)
                      n174 = call "compliancevi3subvi.vi"("compliance (A)"=w454, "start"=w450, "compliance (V)"=w452, "total points"=w453, "step"=w448, "Mode"=w458) -> ("total points 2"=w451:u16, "compliance"=w449:dbl)  [unwired: 1 in, 1 out]
                      n175 = call "HP415xA _Config-Sweep-Secondary Sour.vi"("compliance"=w449, "step"=w448, "error in (no error)"=w456, "total points"=w451, "start"=w450, "VISA session"=w457) -> ("error out"=w455:errorcluster)  [unwired: 1 in]
                      n176 = local write "error?"(w455) -> ()
                    }
                  }
                }
                frame True {
                  n177 = local read "Mode"() -> (w466:u16)
                  n178 = call "compliancevi3subvi.vi"("compliance (A)"=w464, "start"=w459, "compliance (V)"=w463, "total points"=w465, "step"=w461, "Mode"=w466) -> ("total points 2"=w460:u16, "compliance"=w462:dbl)  [unwired: 1 in, 1 out]
                  n179 = call "HP415xA _Config-Sweep-Secondary Sour.vi"("compliance"=w462, "step"=w461, "error in (no error)"=w468, "total points"=w460, "start"=w459, "VISA session"=w469) -> ("error out"=w467:errorcluster)  [unwired: 1 in]
                  n180 = local write "error?"(w467) -> ()
                }
              }
            }
          }
        }
        frame True {
          w478 = u16 2 items=["disabled", "Var1", "Var2", "Var1'", "Constant"] ("Function 2")
          n181 = local read "error?"() -> (w480:errorcluster)
          n182 = local read "Mode"() -> (w488:u16)
          n183 = local read "Function 2"() -> (w479:u16)
          n184 = call "compliancesubvi2.vi"("compliance (V)"=w487, "Mode"=w488, "compliance (A)"=w486) -> ("compliance"=w489:dbl)  [unwired: 3 in, 1 out]
          n185 = call "HP415xA _Config-Sweep-Primary Sour.vi"("step (linear only)"=w483, "stop"=w482, "start"=w481, "compliance"=w489, "error in (no error)"=w480, "sweep mode"=w484, "sweep spacing (linear: 0)"=w485, "VISA session"=w470) -> ("error out"=w471:errorcluster)  [unwired: 2 in]
          n186 = Equal?(x=w479, y=w478) -> (x = y?=w477:bool)
          n187 = case shown="True" w477 {
            tunnel: w476 -> [w495 w539]
            tunnel: w475 -> [w496 w538]
            tunnel: w474 -> [w493 w535]
            tunnel: w473 -> [w494 w537]
            tunnel: w472 -> [w492 w533]
            tunnel: w471 -> [w491 w542]
            tunnel: w470 -> [w490 w540]
            frame False {
              w499 = u16 2 items=["disabled", "Var1", "Var2", "Var1'", "Constant"] ("Function 2")
              n188 = local read "Function 3"() -> (w498:u16)
              n189 = Equal?(x=w498, y=w499) -> (x = y?=w497:bool)
              n190 = case shown="True" w497 {
                tunnel: w496 -> [w504 w522]
                tunnel: w495 -> [w505 w523]
                tunnel: w494 -> [w502 w528]
                tunnel: w493 -> [w503 w525]
                tunnel: w492 -> [w501 w524]
                tunnel: w491 -> [w506 w531]
                tunnel: w490 -> [w500 w529]
                frame False {
                  w509 = u16 2 items=["disabled", "Var1", "Var2", "Var1'", "Constant"] ("Function 2")
                  n191 = local read "Function 4"() -> (w508:u16)
                  n192 = Equal?(x=w508, y=w509) -> (x = y?=w507:bool)
                  n193 = case shown="True" w507 {
                    tunnel: w506 -> [w510 w521]
                    tunnel: w505 -> [_ w511]
                    tunnel: w504 -> [_ w512]
                    tunnel: w503 -> [_ w513]
                    tunnel: w502 -> [_ w518]
                    tunnel: w501 -> [_ w515]
                    tunnel: w500 -> [_ w519]
                    frame False {
                      n194 = local write "error?"(w510) -> ()
                    }
                    frame True {
                      n195 = local read "Mode 4"() -> (w517:u16)
                      n196 = call "compliancevi3subvi.vi"("compliance (A)"=w511, "start"=w513, "compliance (V)"=w512, "total points"=w518, "step"=w515, "Mode"=w517) -> ("total points 2"=w514:u16, "compliance"=w516:dbl)  [unwired: 1 in, 1 out]
                      n197 = call "HP415xA _Config-Sweep-Secondary Sour.vi"("compliance"=w516, "step"=w515, "error in (no error)"=w521, "total points"=w514, "start"=w513, "VISA session"=w519) -> ("error out"=w520:errorcluster)  [unwired: 1 in]
                      n198 = local write "error?"(w520) -> ()
                    }
                  }
                }
                frame True {
                  n199 = local read "Mode 3"() -> (w532:u16)
                  n200 = call "compliancevi3subvi.vi"("compliance (A)"=w523, "start"=w525, "compliance (V)"=w522, "total points"=w528, "step"=w524, "Mode"=w532) -> ("total points 2"=w527:u16, "compliance"=w526:dbl)  [unwired: 1 in, 1 out]
                  n201 = call "HP415xA _Config-Sweep-Secondary Sour.vi"("compliance"=w526, "step"=w524, "error in (no error)"=w531, "total points"=w527, "start"=w525, "VISA session"=w529) -> ("error out"=w530:errorcluster)  [unwired: 1 in]
                  n202 = local write "error?"(w530) -> ()
                }
              }
            }
            frame True {
              n203 = local read "Mode 2"() -> (w543:u16)
              n204 = call "compliancevi3subvi.vi"("compliance (A)"=w539, "start"=w535, "compliance (V)"=w538, "total points"=w537, "step"=w533, "Mode"=w543) -> ("total points 2"=w536:u16, "compliance"=w534:dbl)  [unwired: 1 in, 1 out]
              n205 = call "HP415xA _Config-Sweep-Secondary Sour.vi"("compliance"=w534, "step"=w533, "error in (no error)"=w542, "total points"=w536, "start"=w535, "VISA session"=w540) -> ("error out"=w541:errorcluster)  [unwired: 1 in]
              n206 = local write "error?"(w541) -> ()
            }
          }
        }
      }
    }
    frame #4 {
      # "This step sets the integration time."
      n207 = local read "VISA session"() -> (w544:refnum<visa-resource-name>)
      n208 = local read "error?"() -> (w548:errorcluster)
      n209 = call "HP415xA _Config-Meas-Timing.vi"("error in (no error)"=w548, "wait time parameter"="wait time parameter", "integration time"="integration time", "VISA session"=w544) -> ("error out"=w547:errorcluster)  [unwired: 2 in]
      n210 = local write "error?"(w547) -> ()
    }
    frame #5 {
      w585 = u32 1 items=["stop  ", "single  ", "single-append  ", "stress start  ", "continuous  ", "standby on  ", "standby off  ", "zero  "] ("function (stop:0)")
      w589 = u16 2 items=["disabled", "Var1", "Var2", "Var1'", "Constant"] ("Function")
      w594 = u16 1 items=["disabled", "Var1", "Var2", "Var1'", "Constant"] ("Function")
      n211 = local read "Function"() -> (w596:u16)
      n212 = local read "Function"() -> (w588:u16)
      n213 = Equal?(x=w596, y=w594) -> (x = y?=w595:bool)
      n214 = Equal?(x=w588, y=w589) -> (x = y?=w587:bool)
      n215 = case shown="False" w595 {
        tunnel: [w862 w877] -> w590
        tunnel: [w863 w876] -> _
        tunnel: w594 -> [w860 _]
        frame False {
          n216 = local read "Function 2"() -> (w864:u16)
          n217 = Equal?(x=w864, y=w860) -> (x = y?=w861:bool)
          n218 = case shown="False" w861 {
            tunnel: [w865 w875] -> w863
            tunnel: [w866 w874] -> w862
            tunnel: w860 -> [w869 _]
            frame False {
              n219 = local read "Function 3"() -> (w868:u16)
              n220 = Equal?(x=w868, y=w869) -> (x = y?=w867:bool)
              n221 = case shown="True" w867 {
                tunnel: [w871 w873] -> w866
                tunnel: [w870 w872] -> w865
                frame False {
                  n222 = local read "Vname 4"() -> (w871:string)
                  n223 = local read "Iname 4"() -> (w870:string)
                }
                frame True {
                  n224 = local read "Vname 3"() -> (w873:string)
                  n225 = local read "Iname 3"() -> (w872:string)
                }
              }
            }
            frame True {
              n226 = local read "Iname 2"() -> (w875:string)
              n227 = local read "Vname 2"() -> (w874:string)
            }
          }
        }
        frame True {
          n228 = local read "Vname"() -> (w877:string)
          n229 = local read "Iname"() -> (w876:string)
        }
      }
      n230 = case shown="False" w587 {
        tunnel: [w804 w857] -> w560
        tunnel: [w803 TRUE ("x = y?")] -> w566
        frame False {
          w807 = u16 2 items=["disabled", "Var1", "Var2", "Var1'", "Constant"] ("Function")
          n231 = local read "Function 2"() -> (w806:u16)
          n232 = Equal?(x=w806, y=w807) -> (x = y?=w805:bool)
          n233 = case shown="True" w805 {
            tunnel: [w809 w847] -> w804
            tunnel: [w808 TRUE ("x = y?")] -> w803
            frame False {
              w812 = u16 2 items=["disabled", "Var1", "Var2", "Var1'", "Constant"] ("Function")
              n234 = local read "Function 3"() -> (w811:u16)
              n235 = Equal?(x=w811, y=w812) -> (x = y?=w810:bool)
              n236 = case shown="True" w810 {
                tunnel: [w817 w837] -> w809
                tunnel: [w813 TRUE ("x = y?")] -> w808
                frame False {
                  w816 = u16 2 items=["disabled", "Var1", "Var2", "Var1'", "Constant"] ("Function")
                  n237 = local read "Function 4"() -> (w815:u16)
                  n238 = Equal?(x=w815, y=w816) -> (x = y?=w814:bool)
                  n239 = case shown="True" w814 {
                    tunnel: ["0" ("Vname 4") w827] -> w817
                    tunnel: [FALSE ("x = y?") TRUE ("x = y?")] -> w813
                    frame False {
                    }
                    frame True {
                      w821 = u16 2 items=["V", "I", "VPulse", "IPulse", "Common"] ("Mode 2")
                      w824 = u16 0 items=["V", "I", "VPulse", "IPulse", "Common"] ("Mode 2")
                      n240 = local read "Mode 4"() -> (w823:u16)
                      n241 = Equal?(x=w824, y=w823) -> (x = y?=w825:bool)
                      n242 = Equal?(x=w823, y=w821) -> (x = y?=w822:bool)
                      n243 = Or(x=w825, y=w822) -> (x .or. y?=w820:bool)
                      n244 = case shown="False" w820 {
                        tunnel: [w828 w829] -> w827
                        frame False {
                          n245 = local read "Iname 4"() -> (w828:string)
                        }
                        frame True {
                          n246 = local read "Vname 4"() -> (w829:string)
                        }
                      }
                    }
                  }
                }
                frame True {
                  w833 = u16 2 items=["V", "I", "VPulse", "IPulse", "Common"] ("Mode 2")
                  w832 = u16 0 items=["V", "I", "VPulse", "IPulse", "Common"] ("Mode 2")
                  n247 = local read "Mode 3"() -> (w831:u16)
                  n248 = Equal?(x=w832, y=w831) -> (x = y?=w835:bool)
                  n249 = Equal?(x=w831, y=w833) -> (x = y?=w834:bool)
                  n250 = Or(x=w835, y=w834) -> (x .or. y?=w830:bool)
                  n251 = case shown="False" w830 {
                    tunnel: [w838 w839] -> w837
                    frame False {
                      n252 = local read "Iname 3"() -> (w838:string)
                    }
                    frame True {
                      n253 = local read "Vname 3"() -> (w839:string)
                    }
                  }
                }
              }
            }
            frame True {
              w841 = u16 2 items=["V", "I", "VPulse", "IPulse", "Common"] ("Mode 2")
              w842 = u16 0 items=["V", "I", "VPulse", "IPulse", "Common"] ("Mode 2")
              n254 = local read "Mode 2"() -> (w843:u16)
              n255 = Equal?(x=w842, y=w843) -> (x = y?=w845:bool)
              n256 = Equal?(x=w843, y=w841) -> (x = y?=w844:bool)
              n257 = Or(x=w845, y=w844) -> (x .or. y?=w840:bool)
              n258 = case shown="True" w840 {
                tunnel: [w848 w849] -> w847
                frame False {
                  n259 = local read "Iname 2"() -> (w848:string)
                }
                frame True {
                  n260 = local read "Vname 2"() -> (w849:string)
                }
              }
            }
          }
        }
        frame True {
          w854 = u16 2 items=["V", "I", "VPulse", "IPulse", "Common"] ("Mode")
          w855 = u16 0 items=["V", "I", "VPulse", "IPulse", "Common"] ("Mode")
          n261 = local read "Mode"() -> (w853:u16)
          n262 = Equal?(x=w853, y=w855) -> (x = y?=w852:bool)
          n263 = Equal?(x=w853, y=w854) -> (x = y?=w851:bool)
          n264 = Or(x=w852, y=w851) -> (x .or. y?=w850:bool)
          n265 = case shown="True" w850 {
            tunnel: [w858 w859] -> w857
            frame False {
              n266 = local read "Iname"() -> (w858:string)
            }
            frame True {
              n267 = local read "Vname"() -> (w859:string)
            }
          }
        }
      }
      n268 = local read "error?"() -> (w577:errorcluster)
      n269 = Unbundle("Y2 axis settings") -> ("Y2 axis on/off"=w569:bool, "MINIMUM"=w582:ext, "MAXIMUM"=w581:ext, "Variable name"=w573:string, "LIN or LOG axis"=w580:string)
      n270 = local read "Var2 step settings"() -> (w592:T5)
      n271 = local read "Var1 sweep settings"() -> (w593:T6)
      n272 = local read "VISA session"() -> (w561:refnum<visa-resource-name>)
      n273 = call "Y1subvi.vi"("MAXIMUM"="MAXIMUM", "Variable name"="Y1 axis", "error in (no error)"=w577, "MINIMUM"="MINIMUM", "LIN or LOG axis"="LIN", "VISA resource name"=w561) -> ("error out"=w578:errorcluster)
      n274 = case shown="False" w569 {
        tunnel: w578 -> [w795 w802]
        tunnel: w561 -> [_ w801]
        tunnel: w582 -> [_ w800]
        tunnel: w581 -> [_ w799]
        tunnel: w573 -> [_ w798]
        tunnel: w580 -> [_ w797]
        tunnel: [w795 w796] -> w579
        frame False {
        }
        frame True {
          n275 = call "Y2subvi.vi"("MAXIMUM"=w799, "Variable name"=w798, "error in (no error)"=w802, "MINIMUM"=w800, "LIN or LOG axis"=w797, "VISA resource name"=w801) -> ("error out"=w796:errorcluster)
        }
      }
      n276 = Unbundle(w592) -> ("total points"=w591:u16)  [unwired: 4 out]
      n277 = Decrement(x=w591) -> (x-1=w551:u16)
      n278 = Unbundle(w593) -> ("start"=w559:dbl)  [unwired: 6 out]
      n279 = call "HP415xA Op-Start-Stop.vi"("error in (no error)"=w579, "function (stop:0)"=w585, "wait until finish"=TRUE, "VISA session"=w561) -> ("error out"=w584:errorcluster)  [unwired: 6 in, 1 out]
      n280 = call "HP415xA Op-Download Trace.vi"("error in (no error)"=w584, "trace (variable) name"=w590, "VISA session"=w561) -> ("error out"=w599:errorcluster, "trace"=w567:dbl[])
      n281 = call "HP415xA Op-Download Trace.vi"("error in (no error)"=w599, "trace (variable) name"="Y1 axis", "VISA session"=w561) -> ("error out"=w574:errorcluster, "trace"=w562:dbl[])
      n282 = case shown="True" w569 {
        tunnel: w574 -> [w780 w788]
        tunnel: w561 -> [_ w787]
        tunnel: w573 -> [_ w786]
        tunnel: [w780 w785] -> w563
        tunnel: w567 -> [w778 w784]
        tunnel: w562 -> [w779 w783]
        tunnel: [w777 w782] -> w570
        tunnel: [dbl[] [] ("trace") w781] -> w568
        frame False {
          n283 = Bundle("trace"=w778, "trace"=w779) -> (w777:cluster{"trace":dbl[], "trace":dbl[]})  [unwired: 1 in]
        }
        frame True {
          n284 = call "HP415xA Op-Download Trace.vi"("error in (no error)"=w788, "trace (variable) name"=w786, "VISA session"=w787) -> ("error out"=w785:errorcluster, "trace"=w781:dbl[])
          n285 = stacked-sequence {
            tunnel: w781 -> [_ w793]
            tunnel: w784 -> [w791 w792]
            tunnel: w783 -> [w790 _]
            tunnel: [w789 _] -> w782
            frame #0 {
              n286 = Bundle("trace"=w791, "trace"=w790) -> (w789:cluster{"trace":dbl[], "trace":dbl[]})  [unwired: 1 in]
            }
            frame #1 {
              n287 = Bundle("trace"=w792, "trace"=w793) -> (→"graphic display 2":cluster{"trace":dbl[], "trace":dbl[]})  [unwired: 1 in]
            }
          }
        }
      }
      "graphic display" <- w570
      n288 = case shown="True" w566 {
        tunnel: w559 -> [_ w702]
        tunnel: w562 -> [w604 w701]
        tunnel: w567 -> [w605 w700]
        tunnel: w551 -> [_ w699]
        tunnel: w561 -> [_ w695]
        tunnel: w563 -> [_ w694]
        tunnel: [w606 w693] -> w565
        tunnel: w560 -> [_ w692]
        tunnel: w560 -> [_ w685]
        tunnel: [dbl[] [] ("trace") w691] -> w564
        tunnel: w558 -> [_ w688]
        tunnel: w557 -> [_ w687]
        tunnel: w556 -> [_ w664]
        tunnel: [_ w637] -> w555
        tunnel: [_ w636] -> w554
        tunnel: w553 -> [_ w666]
        tunnel: w552 -> [_ w665]
        tunnel: w551 -> [_ _]
        tunnel: w550 -> [_ _]
        tunnel: w549 -> [_ w647]
        frame False {
          n289 = Build Array(w605, w604) -> (w601:dbl[][])
          n290 = local read "error? 2"() -> (w606:errorcluster)
          n291 = call-poly <vilib>:"Write To Spreadsheet File.vi"("transpose? (no:F)"=TRUE ("append to file? (new file:F)"), "format (%.3f)"="%.5e", "2D data"=w601) -> ()  [unwired: 5 in, 1 out]
        }
        frame True {
          (unwired) "\r"
          w658 = "\r"
          # "Find Smallest Vd Value"
          # "Picks linear Id based on Smallest Vd"
          # "Dielectric"
          # "Data Values"
          # "Headers"
          n292 = call "HP415xA Op-Download Trace.vi"("error in (no error)"=w694, "trace (variable) name"=w692, "VISA session"=w695) -> ("error out"=w693:errorcluster, "trace"=w691:dbl[])
          n293 = Initialize Array("") -> (w668:string[])  [unwired: 1 in]
          n294 = for {
            N: w699 -> [w703]
            shift-right: [w720] -> w637
            shift-left: w700 -> [w716]
            tunnel: w702 -> [w722]
            tunnel: [w721] -> _ mode=indexing
            shift-right: [w717] -> w636
            shift-left: w701 -> [w719]
            tunnel: [w718] -> w640 mode=indexing
            shift-right: [w713] -> w682
            shift-left: w691 -> [w715]
            tunnel: w685 -> [_]
            tunnel: [w707] -> w642 mode=indexing
            shift-right: [w706] -> w672
            shift-left: w668 -> [w705]
            tunnel: [w703] -> _ mode=indexing
            # "Cuts data at each new loop"
            # "Id Data"
            # "Vd Data"
            # "Vg Data"
            n295 = Search 1D Array(1D array=w716, element=w722, start index (0)=1) -> (index of element=w714:i32)
            n296 = Split 1D Array(array=w715, index=w714) -> (first subarray=w711:dbl[], second subarray=w713:dbl[])
            n297 = Split 1D Array(array=w716, index=w714) -> (first subarray=w721:dbl[], second subarray=w720:dbl[])
            n298 = Split 1D Array(array=w719, index=w714) -> (first subarray=w718:dbl[], second subarray=w717:dbl[])
            n299 = Array Size(array=w711) -> (size(s)=w710:i32)
            n300 = Decrement(x=w710) -> (x-1=w709:i32)
            n301 = Array Subset(array=w711, index=w709) -> (w712:dbl[])  [unwired: 1 in]
            n302 = Number To Exponential String(number=w712) -> (E-format string=w708:string[])  [unwired: 3 in]
            n303 = Build Array (concatenate)("Id", w705) -> (w706:string[])
            n304 = Concatenate Strings(w708) -> (w707:string)
          }
          n305 = local read "Temp (K)"() -> (w614:dbl)
          n306 = Fract/Exp String To Number(string=w665) -> (number=w645:dbl)  [unwired: 3 in, 1 out]
          n307 = Fract/Exp String To Number(string=w666) -> (number=w646:dbl)  [unwired: 3 in, 1 out]
          n308 = local read "Temp (K)"() -> (w634:dbl)
          n309 = local read "NumPts"() -> (w644:dbl)
          n310 = local read "NumPts"() -> (w635:dbl)
          n311 = Fract/Exp String To Number(string=w647) -> (number=w638:dbl)  [unwired: 3 in, 1 out]
          n312 = Array Size(array=w682) -> (size(s)=w683:i32)
          n313 = call "STS Calculator.vi"("NumPts"=w635, "Saturation Id"=w636, "Vg Column"=w637) -> ("Sub Threshold Swing"=w628:dbl)  [unwired: 6 in, 2 out]
          n314 = call "Mobility-Vt Calculator_Saturation.vi"("Vg Column"=w637, "Sat Id Column"=w636, "NumPts"=w635, "Length"=w645, "Width"=w646, "Dielectric Thickness"=w638) -> ("Check Cluster"=w624:T7, "Log Plot"=w616:cluster{dbl[], dbl[]}, "Mobility-Sat"=w633:dbl, "VT-Sat"=w629:dbl, "XY Graph-Sat"=w617:cluster{dbl[], dbl[]}[], "Off I-Sat"=w630:dbl, "On/Off I-Sat"=w631:dbl)  [unwired: 1 in, 2 out]
          n315 = local write "Check Cluster"(w624) -> ()
          n316 = Decrement(x=w683) -> (x-1=w681:i32)
          n317 = call "Trap Density_VT.vi"("VT"=w629, "Dielectric"=w638) -> ("Trap Density-VT"=w627:dbl)
          n318 = call "Trap Density_STS.vi"("Temp (T) [K]"=w634, "S.T.S. (S)"=w628, "Dielectric"=w638) -> ("Trap Density (N)"=w626:dbl)  [unwired: 8 in]
          n319 = Array Subset(array=w682, index=w681) -> (w680:dbl[])  [unwired: 1 in]
          n320 = Number To Exponential String(number=w680) -> (E-format string=w676:string[])  [unwired: 3 in]
          n321 = Build Array("Sample Temp (K):", "", "Mobility-Sat (cm^2/Vs):", "Mobility-Lin (cm^2/Vs):", "On/Off I-Sat:", "Off I-Sat (A):", "Vt-Sat (V):", "STS-Sat (V/decade):", "Trap Density-VT (Traps/Vcm^2):", "Trap Density-STS (Traps/Vcm^2):") -> (w662:string[])
          n322 = Build Array (concatenate)(w637, w640, w636) -> (w698:dbl[][])
          n323 = Concatenate Strings(w676) -> (w641:string)
          n324 = Build Array (concatenate)(w642, w641) -> (w639:string[])
          n325 = Fract/Exp String To Number(string=w639) -> (number=w622:dbl[])  [unwired: 3 in, 1 out]
          n326 = local write "Test Array"(w622) -> ()
          n327 = Build Array (concatenate)(w640, w636) -> (w620:dbl[][])
          n328 = Build Array("Vg", "Id") -> (w673:string[])
          n329 = Absolute Value(x=w622) -> (abs(x)=w623:dbl[])
          n330 = Insert Into Array(array=w673, index=2, new element=w672) -> (w671:string[])
          n331 = Array Max & Min(array=w623) -> (min index (indices)=w619:i32)  [unwired: 3 out]
          n332 = Index Array(array=w622, index=w619) -> (element=w621:dbl)
          n333 = Build Array (concatenate)("Vd=", w642, w641) -> (w679:string[])
          n334 = Transpose 2D Array(2D array=w698) -> (transposed array=w696:dbl[][])
          n335 = Index Array(array=w620, index (row)=w619) -> (element=w618:dbl[])  [unwired: 1 in]
          n336 = call "Mobility-Vt Calculator_Linear.vi"("Vg Column"=w637, "Vd"=w621, "Lin Id Column"=w618, "NumPts"=w644, "Length"=w645, "Width"=w646, "Dielectric Thickness"=w638) -> ("Mobility-Lin"=w632:dbl)  [unwired: 4 in, 4 out]
          n337 = Build Array(w614, w633, w632, w631, w630, w629, w628, w627, w626) -> (w661:dbl[])
          n338 = Number To Exponential String(number=w661) -> (E-format string=w613:string[])  [unwired: 3 in]
          n339 = Bundle("Mobility-Sat"=w633, "Mobility-Lin"=w632, "On/Off I-Sat"=w631, "Off I-Sat"=w630, "VT-Sat"=w629, "Sub Threshold Swing"=w628, "Trap Density-VT"=w627, "Trap Density (N)"=w626) -> (w625:T8)  [unwired: 1 in]
          n340 = local write "Output"(w625) -> ()
          n341 = Insert Into Array(array=w613, index=1, new element="") -> (w610:string[])
          n342 = Build Array(w662, w610) -> (w609:string[][])
          n343 = Transpose 2D Array(2D array=w609) -> (transposed array=w608:string[][])
          "Test Array 2" <- w608
          n344 = Array To Spreadsheet String(array=w679, 3:"%s") -> (spreadsheet string=w684:string)  [unwired: 1 in]
          n345 = Array To Spreadsheet String(array=w671, 3:"%s") -> (spreadsheet string=w677:string)  [unwired: 1 in]
          n346 = Array To Spreadsheet String(array=w608, 3:"%s") -> (spreadsheet string=w659:string)  [unwired: 1 in]
          n347 = Array To Spreadsheet String(array=w696, 3:"%.5e" ("format string")) -> (spreadsheet string=w686:string)  [unwired: 1 in]
          n348 = Concatenate Strings(w688, w658, w687, w658, w664, w659, w658, w684, w677, w686, "\r") -> (w690:string)
          n349 = local read "Input Path"() -> (w648:path)
          n350 = local write "XY Graph"(w617) -> ()
          n351 = local write "Log Plot"(w616) -> ()
          n352 = call <vilib>:"Write Characters To File.vi"("append to file? (new file:F)"=TRUE, "character string"=w690, "file path (dialog if empty)"=w648) -> ("new file path (Not A Path if cancelled)"=w656:path)  [unwired: 2 in]
          n353 = local write "Output Path"(w656) -> ()
        }
      }
      n354 = case shown="True" w569 {
        tunnel: w551 -> [_ w729]
        tunnel: w566 -> [_ w730]
        tunnel: w567 -> [_ w728]
        tunnel: w559 -> [_ w727]
        tunnel: w568 -> [_ w726]
        tunnel: w564 -> [_ w725]
        tunnel: w560 -> [_ w724]
        frame False {
        }
        frame True {
          n355 = case shown="True" w730 {
            tunnel: w729 -> [_ w746]
            tunnel: w728 -> [w734 w761]
            tunnel: w727 -> [_ w760]
            tunnel: w726 -> [w735 w759]
            tunnel: w725 -> [_ w758]
            tunnel: w724 -> [_ w741]
            frame False {
              n356 = Build Array(w734, w735) -> (w733:dbl[][])
              n357 = call-poly <vilib>:"Write To Spreadsheet File.vi"("transpose? (no:F)"=TRUE, "format (%.3f)"="%.5e", "2D data"=w733) -> ()  [unwired: 5 in, 1 out]
            }
            frame True {
              n358 = for {
                N: w746 -> [_]
                shift-right: [w772] -> w757
                shift-left: w761 -> [w773]
                tunnel: w760 -> [w775]
                tunnel: [w771] -> _ mode=indexing
                shift-right: [w768] -> w755
                shift-left: w759 -> [w770]
                tunnel: [w769] -> w756 mode=indexing
                shift-right: [w765] -> w750
                shift-left: w758 -> [w766]
                tunnel: [w762] -> w747 mode=indexing
                n359 = Search 1D Array(1D array=w773, element=w775, start index (0)=1) -> (index of element=w767:i32)
                n360 = Split 1D Array(array=w773, index=w767) -> (first subarray=w771:dbl[], second subarray=w772:dbl[])
                n361 = Split 1D Array(array=w770, index=w767) -> (first subarray=w769:dbl[], second subarray=w768:dbl[])
                n362 = Split 1D Array(array=w766, index=w767) -> (first subarray=w763:dbl[], second subarray=w765:dbl[])
                n363 = Index Array(array=w763, index=1) -> (element=w762:dbl)
              }
              n364 = Build Array (concatenate)(w757, w756, w755) -> (w754:dbl[][])
              n365 = Index Array(array=w750, index=1) -> (element=w748:dbl)
              n366 = Transpose 2D Array(2D array=w754) -> (transposed array=w753:dbl[][])
              n367 = Insert Into Array(array=w747, index=w746, new element=w748) -> (w745:dbl[])
              n368 = Array To Spreadsheet String(delimiter (Tab)=",", array=w745, 3:"%.5e" ("format string")) -> (spreadsheet string=w739:string)
              n369 = Array To Spreadsheet String(delimiter (Tab)=",", array=w753, 3:"%.5e" ("format string")) -> (spreadsheet string=w737:string)
              n370 = Concatenate Strings(w741, "," ("string")) -> (w740:string)
              n371 = Concatenate Strings(w740, w739) -> (w738:string)
              n372 = Concatenate Strings(w738, w737) -> (w736:string)
              n373 = call <vilib>:"Write Characters To File.vi"("character string"=w736) -> ()  [unwired: 4 in, 1 out]
            }
          }
        }
      }
      n374 = call "HP415xA Sys-Error Query.vi"("VISA session"=w561, "error in (no error)"=w565) -> ("error out"=w597:errorcluster)  [unwired: 2 in, 1 out]
      n375 = call "HP415xA  Close.vi"("error in (no error)"=w597, "VISA session"=w561) -> ("error out"=w598:errorcluster)
      n376 = local write "error?"(w598) -> ()
    }
  }
